vi "Pump Pause Selection.vi"(8 "error in (no error)":errorcluster, 11 "Pump Settings In":T1 {"Masterflex"."Pump Number" min=1.0 max=20.0 step=1.0; "Ismatech"."Pump Number" min=1.0 max=20.0 step=1.0; "ASIA Pump C"."channel" min=-1 max=1 step=1}) -> (0 "error out":errorcluster, 1 "Connection Error":bool, 3 "Pump Settings Out":T1 {"Masterflex"."Pump Number" min=1.0 max=20.0 step=1.0; "Ismatech"."Pump Number" min=1.0 max=20.0 step=1.0; "ASIA Pump C"."channel" min=-1 max=1 step=1})   [LabVIEW 2018, in "Pump Module.lvlib" / "Pump Module Engine.lvlib"]
uses:
  Pump Module Engine.lvlib
  Pump Settings Cluster.ctl
  Measure Instrument/PID 2 Output Enum.ctl
  Masterflex 7550-30/Controls/Settings Cluster.ctl
  Ismatec ISM 831C/Controls/Ismatech Settings Cluster.ctl
  VICI M50 Party Mode/Settings Cluster.ctl
  Tacmina QI/Tacmina QI DAQ Setting.ctl
  KNF Pump/Settings Cluster plus SIMDOS.ctl
  ASIA Pump/Pump Settings.ctl
  FLOM Pump/Settings Cluster.ctl
  SSI PR Class/SSI PR or LD Settings Cluster.ctl
  Masterflex 75211/Masterflex 75211 DAQ Setting.ctl
  Ismatec ISM 831C/Ismatec ISM 831C.lvlib
  Masterflex 7550-30/Masterflex 7550-30.lvlib
  VICI M50 Party Mode/VICI M6 M50 Party Mode.lvlib
  Tacmina QI/Tacmina QI.lvlib
  KNF Pump/KNF SIMDOS.lvlib
  ASIA Pump.lvlib
  FLOM Pump/FLOM Pump.lvlib
  SSI PR Class/SSI PR or LD Pump.lvlib
  Masterflex 75211/Masterflex 75211.lvlib
  SSI PR Class/SSI P40 Pump.lvlib
  Pump Module.lvlib
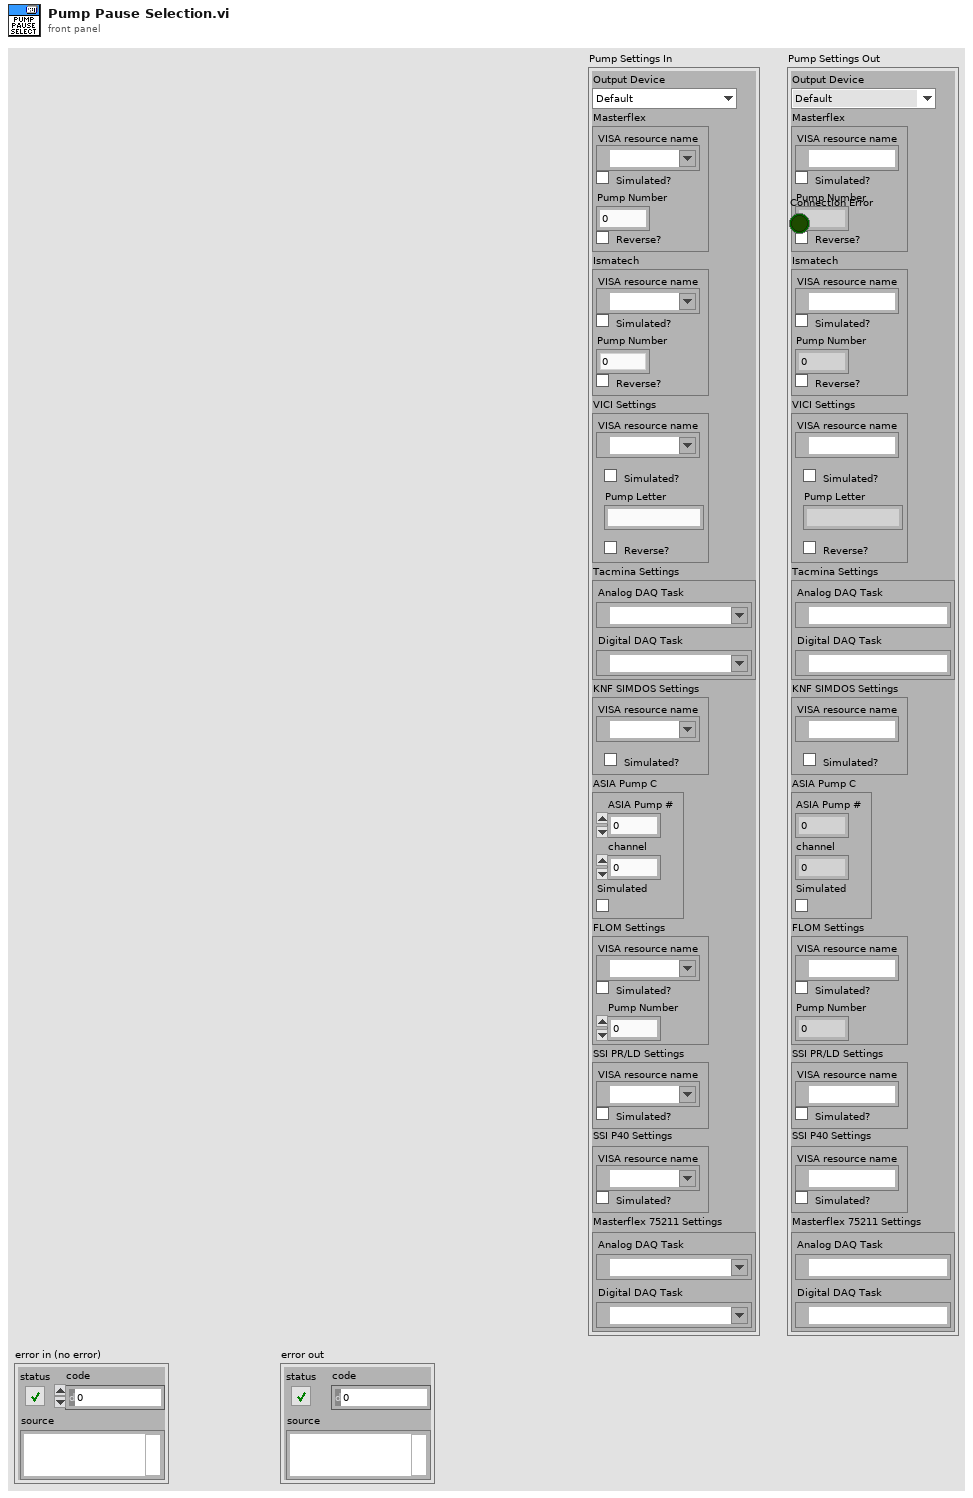
[diagram p1: front panel]
types:
  T1 = typedef "Pump Module.lvlib/Pump Settings Cluster.ctl" = cluster{"Output Device":T2, "Masterflex":T3, "Ismatech":T4, "VICI Settings":T5, "Tacmina Settings":T6, "KNF SIMDOS Settings":T7, "ASIA Pump C":T8, "FLOM Settings":T9, "SSI PR/LD Settings":T10, "SSI P40 Settings":T10, "Masterflex 75211 Settings":T11}
  T2 = typedef "PID 2 Output Enum.ctl" = enum16{"Default", "Ismatec ISM 831C", "Masterflex 7550-30", "VICI", "Tacmina QI", "KNF SIMDOS", "ASIA Type C", "FLOM UI-22-11", "SSI PR/LD", "SSI P40", "Masterflex 75211-70"}
  T3 = typedef "Masterflex 7550-30.lvlib/Settings Cluster.ctl" = cluster{"VISA resource name":refnum<visa-resource-name>, "Simulated?":bool, "Pump Number":dbl, "Reverse?":bool}
  T4 = typedef "Ismatec ISM 831C.lvlib/Ismatech Settings Cluster.ctl" = cluster{"VISA resource name":refnum<visa-resource-name>, "Simulated?":bool, "Pump Number":dbl, "Reverse?":bool}
  T5 = typedef "VICI M6 M50 Party Mode.lvlib/Settings Cluster.ctl" = cluster{"VISA resource name":refnum<visa-resource-name>, "Simulated?":bool, "Pump Letter":string, "Reverse?":bool}
  T6 = typedef "Tacmina QI.lvlib/Tacmina QI DAQ Setting.ctl" = cluster{"Analog DAQ Task":refnum<k21>, "Digital DAQ Task":refnum<k21>}
  T7 = typedef "KNF SIMDOS.lvlib/Settings Cluster plus SIMDOS.ctl" = cluster{"VISA resource name":refnum<visa-resource-name>, "Simulated?":bool}
  T8 = typedef "ASIA Pump.lvlib/Pump Settings.ctl" = cluster{"ASIA Pump #":i32, "channel":i32, "Simulated":bool}
  T9 = typedef "FLOM Pump.lvlib/Settings Cluster.ctl" = cluster{"VISA resource name":refnum<visa-resource-name>, "Simulated?":bool, "Pump Number":dbl}
  T10 = typedef "SSI PR or LD Pump.lvlib/SSI PR or LD Settings Cluster.ctl" = cluster{"VISA resource name":refnum<visa-resource-name>, "Simulated?":bool}
  T11 = typedef "Masterflex 75211.lvlib/Masterflex 75211 DAQ Setting.ctl" = cluster{"Analog DAQ Task":refnum<k21>, "Digital DAQ Task":refnum<k21>}
  T12 = typedef "SSI P40 Pump.lvlib/SSI P40 Settings Cluster.ctl" = cluster{"VISA resource name":refnum<visa-resource-name>, "Simulated?":bool}
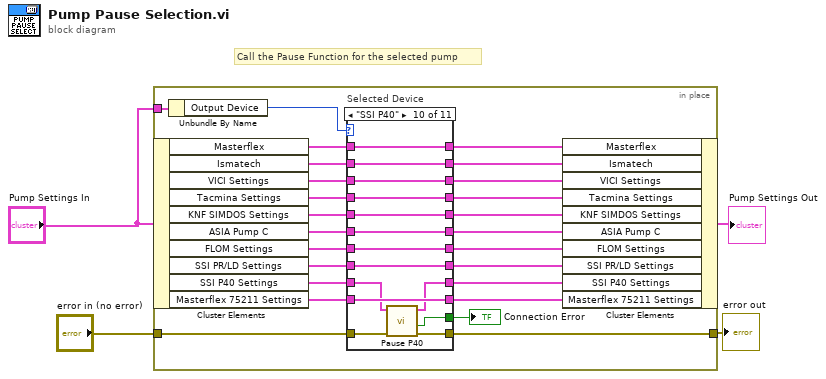
[diagram p0: block diagram]
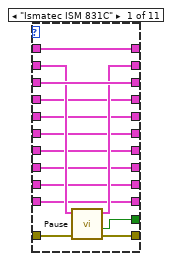
[diagram p2: hidden frame]
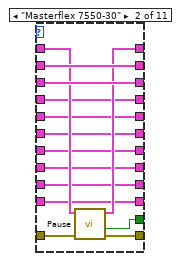
[diagram p3: hidden frame]
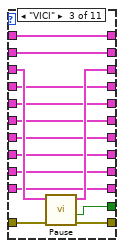
[diagram p4: hidden frame]
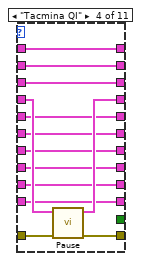
[diagram p5: hidden frame]
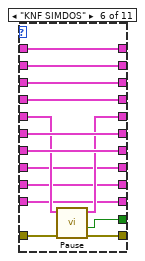
[diagram p7: hidden frame]
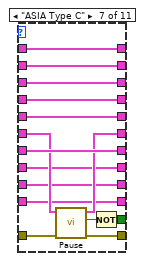
[diagram p8: hidden frame]
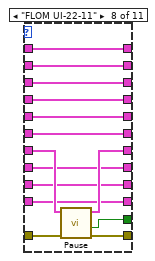
[diagram p9: hidden frame]
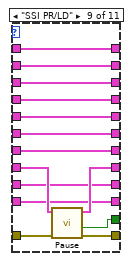
[diagram p10: hidden frame]
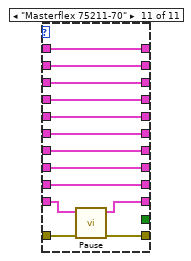
[diagram p11: hidden frame]
diagram:
  # "Call the Pause Function for the selected pump"
  n1 = in-place {
    in-place-border: "error in (no error)" -> [w29]
    in-place-border: [w28] -> w3
    in-place-border: "Pump Settings In" -> [w10]
    n2 = in-place-cluster #1("Pump Settings In") -> ("Masterflex"=w26:T3, "Ismatech"=w25:T4, "VICI Settings"=w24:T5, "Tacmina Settings"=w23:T6, "KNF SIMDOS Settings"=w22:T7, "ASIA Pump C"=w21:T8, "FLOM Settings"=w20:T9, "SSI PR/LD Settings"=w19:T10, "SSI P40 Settings"=w5:T10, "Masterflex 75211 Settings"=w8:T11)
    n3 = Unbundle By Name(w10) -> ("Output Device"=w9:T2)
    n4 = case "Selected Device" shown="\"SSI P40\"" w9 {
      tunnel: w26 -> [w43 w55 w70 w83 w95 w109 w124 w138 w152 w166 w179]
      tunnel: [w43 w54 w70 w83 w95 w109 w124 w138 w152 w166 w179] -> w18
      tunnel: w25 -> [w41 w57 w71 w84 w94 w108 w123 w137 w151 w165 w178]
      tunnel: [w39 w53 w67 w79 w91 w102 w117 w131 w144 w156 w168] -> w28
      tunnel: [w40 w57 w71 w84 w94 w108 w123 w137 w151 w165 w178] -> w17
      tunnel: w24 -> [w42 w56 w69 w82 w93 w107 w122 w136 w150 w164 w177]
      tunnel: [w42 w56 w68 w82 w93 w107 w122 w136 w150 w164 w177] -> w16
      tunnel: w23 -> [w37 w51 w65 w81 w92 w106 w121 w135 w149 w163 w176]
      tunnel: [w37 w51 w65 w80 w92 w106 w121 w135 w149 w163 w176] -> w15
      tunnel: w29 -> [w38 w52 w66 w78 w91 w103 w118 w132 w145 w157 w169]
      tunnel: [w36 w50 w64 w77 w90 w101 w120 w134 w148 w162 w175] -> w14
      tunnel: w22 -> [w36 w50 w64 w77 w90 w100 w120 w134 w148 w162 w175]
      tunnel: [w35 w49 w63 w76 w89 w105 w116 w133 w147 w161 w174] -> w13
      tunnel: w21 -> [w35 w49 w63 w76 w89 w105 w115 w133 w147 w161 w174]
      tunnel: [w34 w48 w62 w75 w88 w104 w119 w129 w146 w160 w173] -> w12
      tunnel: w20 -> [w34 w48 w62 w75 w88 w104 w119 w130 w146 w160 w173]
      tunnel: [w33 w47 w61 w74 w87 w99 w114 w128 w142 w159 w172] -> w11
      tunnel: w19 -> [w33 w47 w61 w74 w87 w99 w114 w128 w143 w159 w172]
      tunnel: [w32 w46 w60 _ _ w98 w112 w127 w141 w155 _] -> w27
      tunnel: w8 -> [w31 w45 w59 w73 w86 w97 w111 w126 w140 w158 w171]
      tunnel: [w31 w45 w59 w73 w86 w97 w111 w126 w140 w158 w170] -> w7
      tunnel: [w30 w44 w58 w72 w85 w96 w110 w125 w139 w154 w167] -> w6
      tunnel: w5 -> [w30 w44 w58 w72 w85 w96 w110 w125 w139 w153 w167]
      frame "Ismatec ISM 831C" {
        n5 = call "Pause.vi"("error in (no error)"=w38, "Ismatech Settings In"=w41) -> ("error out"=w39:errorcluster, "Connection Error"=w32:bool, "Ismatech Settings Out"=w40:T4)  [unwired: 7 in]
      }
      frame "Masterflex 7550-30" {
        n6 = call "Pause.vi"("error in (no error)"=w52, "Masterflex Settings in"=w55) -> ("error out"=w53:errorcluster, "Connection Error"=w46:bool, "Masterflex Settings out"=w54:T3)  [unwired: 7 in]
      }
      frame "VICI" {
        n7 = call "Pause.vi"("error in (no error)"=w66, "VICI Settings In"=w69) -> ("error out"=w67:errorcluster, "Connection Error"=w60:bool, "VICI Settings Out"=w68:T5)  [unwired: 7 in]
      }
      frame "Tacmina QI" {
        n8 = call "Pause.vi"("error in"=w78, "Tacmina Settings in"=w81) -> ("error out"=w79:errorcluster, "Tacmina Settings out"=w80:T6)  [unwired: 8 in]
      }
      frame "Default", Default {
      }
      frame "KNF SIMDOS" {
        n9 = call "Pause.vi"("error in (no error)"=w103, "KNF Settings In"=w100) -> ("error out"=w102:errorcluster, "Connection Error"=w98:bool, "KNF Settings Out"=w101:T7)  [unwired: 7 in]
      }
      frame "ASIA Type C" {
        n10 = call "Pause.vi"("error in (no error)"=w118, "ASIA Pump C Settings in"=w115) -> ("error out"=w117:errorcluster, "Task Completed"=w113:bool, "ASIA Pump C Settings out"=w116:T8)  [unwired: 7 in]
        n11 = Not(x=w113) -> (.not. x?=w112:bool)
      }
      frame "FLOM UI-22-11" {
        n12 = call "Pause.vi"("error in (no error)"=w132, "FLOM Settings in"=w130) -> ("error out"=w131:errorcluster, "Connection Error"=w127:bool, "FLOM Settings out"=w129:T9)  [unwired: 7 in]
      }
      frame "SSI PR/LD" {
        n13 = call "Pause.vi"("error in (no error)"=w145, "SSI PR Settings In"=w143) -> ("error out"=w144:errorcluster, "Connection Error"=w141:bool, "SSI PR Settings Out"=w142:T10)  [unwired: 6 in]
      }
      frame "SSI P40" {
        n14 = call "Pause P40.vi"("error in (no error)"=w157, "SSI P40 Settings In"=w153) -> ("error out"=w156:errorcluster, "Connection Error"=w155:bool, "SSI P40 Settings Out"=w154:T12)  [unwired: 7 in]
      }
      frame "Masterflex 75211-70" {
        n15 = call "Pause.vi"("error in"=w169, "Masterflex 75211 Settings"=w171) -> ("error out"=w168:errorcluster, "Masterflex 75211 Settings"=w170:T11)  [unwired: 8 in]
      }
    }
    "Connection Error" <- w27
    n16 = in-place-cluster #1("Masterflex"=w18, "Ismatech"=w17, "VICI Settings"=w16, "Tacmina Settings"=w15, "KNF SIMDOS Settings"=w14, "ASIA Pump C"=w13, "FLOM Settings"=w12, "SSI PR/LD Settings"=w11, "SSI P40 Settings"=w6, "Masterflex 75211 Settings"=w7) -> (→"Pump Settings Out":T1)
  }
  "error out" <- w3
